vi "uActor_Core.vi"(8 "error in (no error)":errorcluster, 11 "uBroker in":refnum<class "uBroker.lvclass">) -> (0 "error out":errorcluster, 3 "uBroker out":refnum<class "uBroker.lvclass">)   [LabVIEW 2023, in "uLib.lvlib" / "uBroker.lvclass"]
uses:
  uBroker.lvclass
  U:/Projects/uLib/Src/uFramework/uActor/uActor.lvclass
  uMsg/uMsg/uMsg.lvclass
  uMsg/uMsg/uMsg.lvclass/uMsg.ctl
  uActor/uActor/uActor.lvclass/uActor.ctl
  uBroker.lvclass/uBroker.ctl
  uData/uData/uData.lvclass/uData.ctl
  uClient/uClient/uClient.lvclass/uClient.ctl
  uClient/uClient_Subscriber/uClient_Subscriber.lvclass/uClient_Subscriber.ctl
  uPolicy/uPolicy/uPolicy.lvclass/uPolicy.ctl
  uSubscription/uSubscription/uSubscription.lvclass/uSubscription.ctl
  uClient/uClient_Publisher/uClient_Publisher.lvclass/uClient_Publisher.ctl
  uNotifyMode/uNotifyMode/uNotifyMode.lvclass/uNotifyMode.ctl
  uTransport/uTransport_uActor/uTransport_uActor.lvclass/uTransport_uActor.ctl
  uTransport/uTransport_Event/uTransport_Event.lvclass/uTransport_Event.ctl
  uTransport/uTransport_Queue/uTransport_Queue.lvclass/uTransport_Queue.ctl
  uData/uData/Get Tag.vi
  uSubscription/uSubscription/uSubscription Destruct.vi
  uSubscription/uSubscription/uSubscription Construct.vi
  uBroker_Fanout.vi
  uClient/uClient_Publisher/uPublisher IsAlive.vi
  uSubscription/uSubscription/uSubscription IsAlive.vi
  uMsg/uMsg/uMsg Send Reply.vi
  uData/uData/Set Tag.vi
  uMsg/uMsg/uMsg Get CMD.vi
  uTransport/uTransport_uActor/uTransport_uActor_SendMsg.vi
  uMsg/uMsg/uMsg Get Payload.vi
  uData/uData/Condition Tag Name.vi
  uClient/uClient/uClient_GetTransport.vi
  uClient/uClient_Subscriber/uSubscriber Get uPolicy.vi
  uPolicy/uPolicy/Read uNotifyMode.vi
  uPolicy/uPolicy/Read uStringManipulation.vi
  uSubscription/uSubscription/uSubscription Update.vi
  uClient/uClient_Publisher/uPublisher GetGUID.vi
  uData/uData/Combine Tags.vi
  uTransport/uTransport/uTransport_SendMsg.vi
  uData/uData/Blank Key Reserved String.vi
  uMsg/uMsg/uMsg Rename CMD.vi
  uNotifyMode/uNotifyMode/uNotify Update.vi
  uMsg/uMsg/uMsg Update Timestamp.vi
  uTransport/uTransport_Event/uTransport_Event_SendMsg.vi
  uTransport/uTransport_Queue/uTransport_Queue_SendMsg.vi
  uClient/uClient_Subscriber/uClient_Subscriber.lvclass
  U:/Projects/uLib/Src/uFramework/uClient/uClient.lvclass
  uClient/uClient_Publisher/uClient_Publisher.lvclass
  uActor/uActor/uActor.lvclass
  uData/uData/uData.lvclass
  uTransport/uTransport/uTransport.lvclass
  uSubscription/uSubscription/uSubscription.lvclass
  uNotifyMode/uNotifyMode/uNotifyMode.lvclass
  uPolicy/uPolicy/uPolicy.lvclass
  uStringManipulation/uStringManipulation/uStringManipulation.lvclass
  uTransport/uTransport_uActor/uTransport_uActor.lvclass
  uTransport/uTransport_Event/uTransport_Event.lvclass
  uTransport/uTransport_Queue/uTransport_Queue.lvclass
  U:/Projects/uLib/Src/uFramework/uTransport/uTransport.lvclass
  U:/Projects/uLib/Src/uFramework/uBroker/uBroker.lvclass
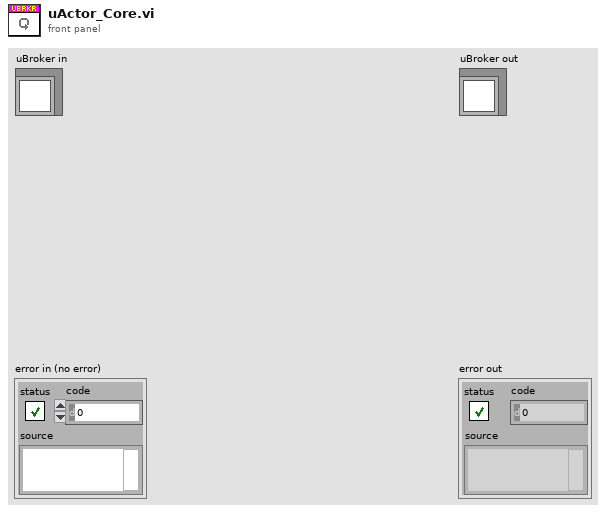
[diagram p1: front panel]
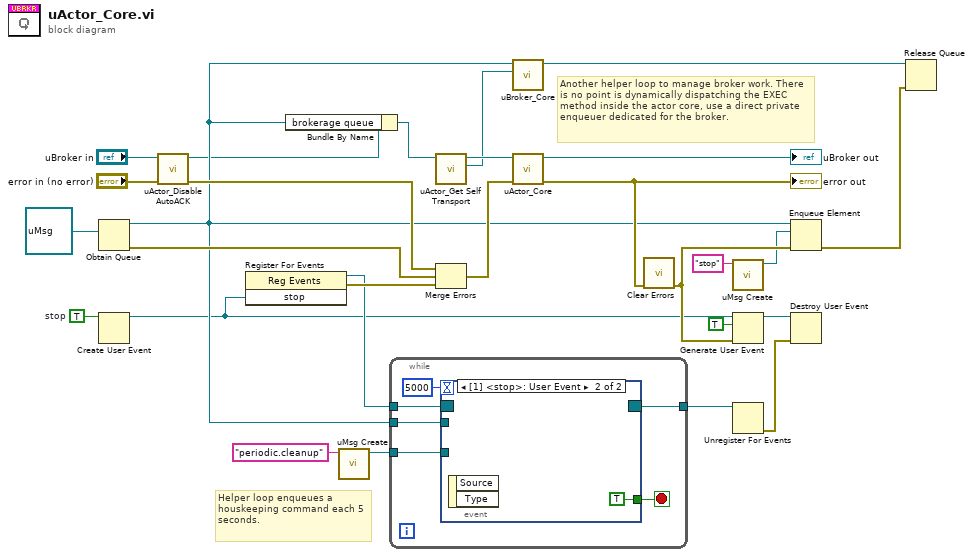
[diagram p0: block diagram]
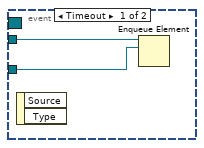
[diagram p2: hidden frame]
diagram:
  w22 = TRUE  # stop
  # "Another helper loop to manage broker work. There is no point is dynamically dispatching the EXEC method inside the actor core, use a direct private enqueuer dedicated for the broker."
  # "Helper loop enqueues a houskeeping command each 5 seconds."
  n1 = Obtain Queue(element data type=refnum<class "uMsg.lvclass"> refnum ("uTransport.lvlib:uMsg.lvclass")) -> (queue out=w11:refnum<queue>, error out=w27:errorcluster)  [unwired: 4 in, 1 out]
  n2 = Create User Event(user event datatype=w22) -> (user event=w10:refnum<user-event>)  [unwired: 1 in, 1 out]
  n3 = call "uActor_Disable AutoACK.vi"("error in (no error)"="error in (no error)", "uActor in"="uBroker in") -> ("error out"=w28:errorcluster, "uActor out"=w1:refnum<class "uBroker.lvclass">)  [unwired: 8 in]
  n4 = register-events(w10) -> (reference out=w21:refnum<event-registration>, error out=w24:errorcluster)  [unwired: 2 in]
  n5 = Bundle By Name(cluster=w1, "brokerage queue"=w11) -> (w9:refnum<class "uBroker.lvclass">)
  n6 = call "uMsg Create.vi"("CMD"="periodic.cleanup") -> ("uMsg out"=w13:refnum<class "uMsg.lvclass">)  [unwired: 9 in, 1 out]
  n7 = while {
    tunnel: w21 -> [w34]
    tunnel: [w33] -> w20
    tunnel: w11 -> [w30]
    tunnel: w13 -> [w29]
    stop <- w31 stop-if-true
    n8 = event shown="[1] <stop>: User Event" {
      selector: w34 -> [_ _]
      dyn-events: [_ _] -> w33
      timeout: 5000 -> [_ _]
      tunnel: [_ TRUE] -> w31
      tunnel: w30 -> [w36 _]
      tunnel: w29 -> [w35 _]
      event Timeout {
        n9 = event-data() -> ()  [unwired: 1 in, 2 out]
        n10 = Enqueue Element(queue=w36, element=w35) -> ()  [unwired: 2 in, 3 out]
      }
      event User Event {
        n11 = event-data() -> ()  [unwired: 1 in, 2 out]
      }
    }
  }
  n12 = call "uActor_Get Self Transport.vi"("uActor in"=w9) -> ("Actor Transport"=w3:refnum<class "uTransport_uActor.lvclass">, "uActor out"=w4:refnum<class "uBroker.lvclass">)  [unwired: 9 in]
  n13 = Merge Errors(w28, w27, w24) -> (w16:errorcluster)
  n14 = call "uBroker_Core.vi"("ActorCore Transport"=w3, "brokerage queue in"=w11) -> ("brokerage queue out"=w6:refnum<queue>)  [unwired: 9 in]
  n15 = call-parent "uActor_Core.vi"("error in (no error)"=w16, "uActor in"=w4) -> ("error out"=w19:errorcluster, "uActor out"=→"uBroker out":refnum<class "uBroker.lvclass">)  [unwired: 8 in]
  "error out" <- w19
  n16 = call <vilib>:"Clear Errors.vi"("error in (no error)"=w19) -> ("error out"=w25:errorcluster)  [unwired: 5 in, 1 out]
  n17 = call "uMsg Create.vi"("CMD"="stop") -> ("uMsg out"=w8:refnum<class "uMsg.lvclass">)  [unwired: 9 in, 1 out]
  n18 = Generate User Event(user event=w10, event data cluster=TRUE ("event data"), error in=w25) -> (user event out=w18:refnum<user-event>)  [unwired: 1 in, 1 out]
  n19 = Unregister For Events(event registration refnum=w20) -> (error out=w17:errorcluster)  [unwired: 1 in]
  n20 = Enqueue Element(queue=w11, element=w8, error in (no error)=w25) -> (error out=w5:errorcluster)  [unwired: 1 in, 2 out]
  n21 = Destroy User Event(user event=w18, error in=w17) -> ()  [unwired: 1 out]
  n22 = Release Queue(queue=w6, error in (no error)=w5) -> ()  [unwired: 1 in, 3 out]
